vi "Draw Shapes.vi"(0 "Picture in":refnum<vi>, 1 "Commands":cluster{"Time (s)":dbl, T2, "Enabled":bool}[](array[cluster]), 3 "Sample Period (s)":dbl=0.02, 5 "Points":cluster{"x":dbl, "y":dbl, "th":dbl}[](array[cluster]), 6 "Path Points MEGA":cluster{"x":dbl, "y":dbl}[][](array[cluster]), 9 "new picture in":picture, 10 "Output Point MEGA":T1(array[cluster]), 11 "Results":T5, 12 "Output Point":T4, 14 "Path Points":cluster{"x":dbl, "y":dbl}[](array[cluster]), 15 "MEGA?":bool) -> (4 "new picture out":picture)   [LabVIEW 2023]
uses:
  Types/Single Cmd Info.ctl
  <vilib>/picture/picture.llb/imagedata.ctl
  Global Settings.vi
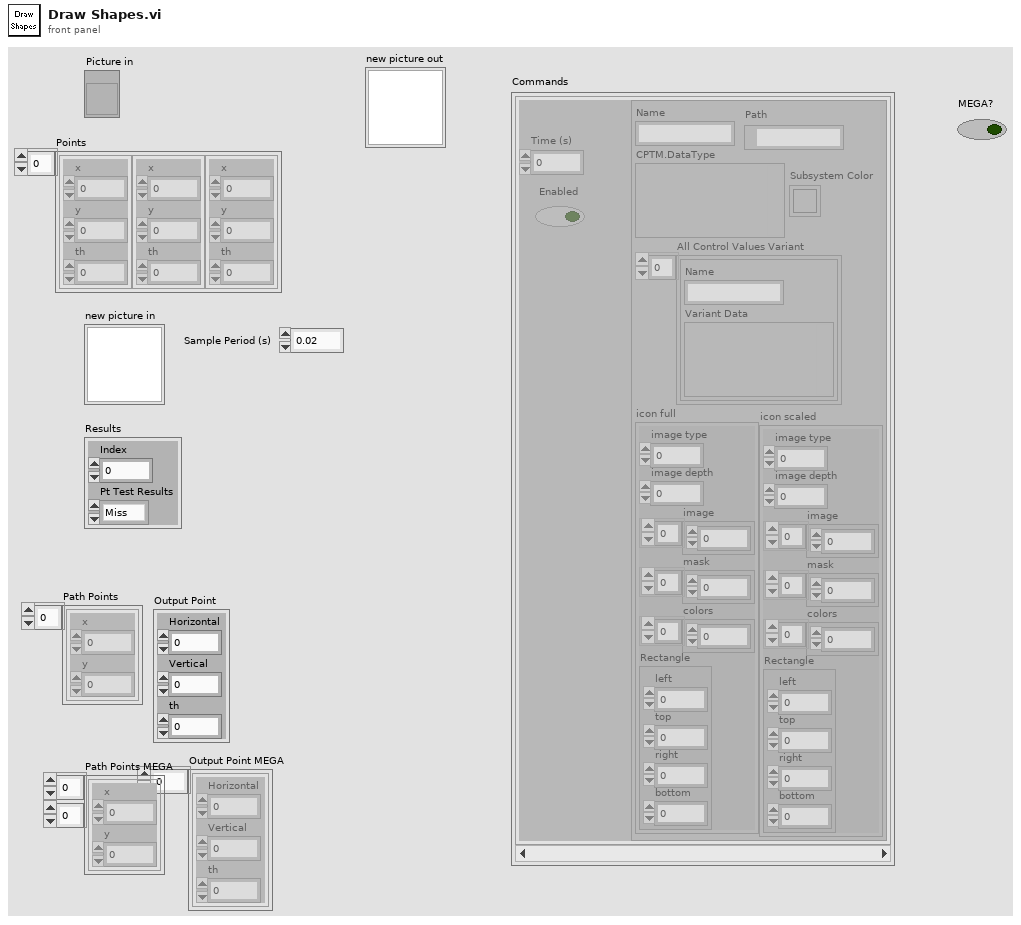
[diagram p1: front panel]
types:
  T1 = cluster{"Horizontal":dbl, "Vertical":dbl, "th":dbl}[]
  T2 = typedef "Single Cmd Info.ctl" = cluster{"Name":string, "CPTM.DataType":variant, "All Control Values Variant":cluster{"Name":string, "Variant Data":variant}[], "icon full":T3, "icon scaled":T3, "Path":path, "Subsystem Color":u32}
  T3 = typedef "imagedata.ctl" = cluster{"image type":i32, "image depth":i32, "image":u8[], "mask":u8[], "colors":u32[], "Rectangle":cluster{"left":i16, "top":i16, "right":i16, "bottom":i16}}
  T4 = cluster{"Horizontal":dbl, "Vertical":dbl, "th":dbl}
  T5 = cluster{"Index":i32, "Pt Test Results":enum16{"Miss", "Rect Hit", "Arrow Hit"}}
  T6 = typedef "LVPositionTypeDef.ctl" = cluster{"Left":i32, "Top":i32}
  T7 = typedef "LVBoundsTypeDef.ctl" = cluster{"Width":u32, "Height":u32}
  T8 = cluster{"left":i16, "top":i16, "right":i16, "bottom":i16}
  T9 = cluster{"Horizontal":dbl, "Vertical":dbl, "Horizontal":dbl, "Vertical":dbl}
  T10 = cluster{i32, "Pt Test Results":enum16{"Miss", "Rect Hit", "Arrow Hit"}}
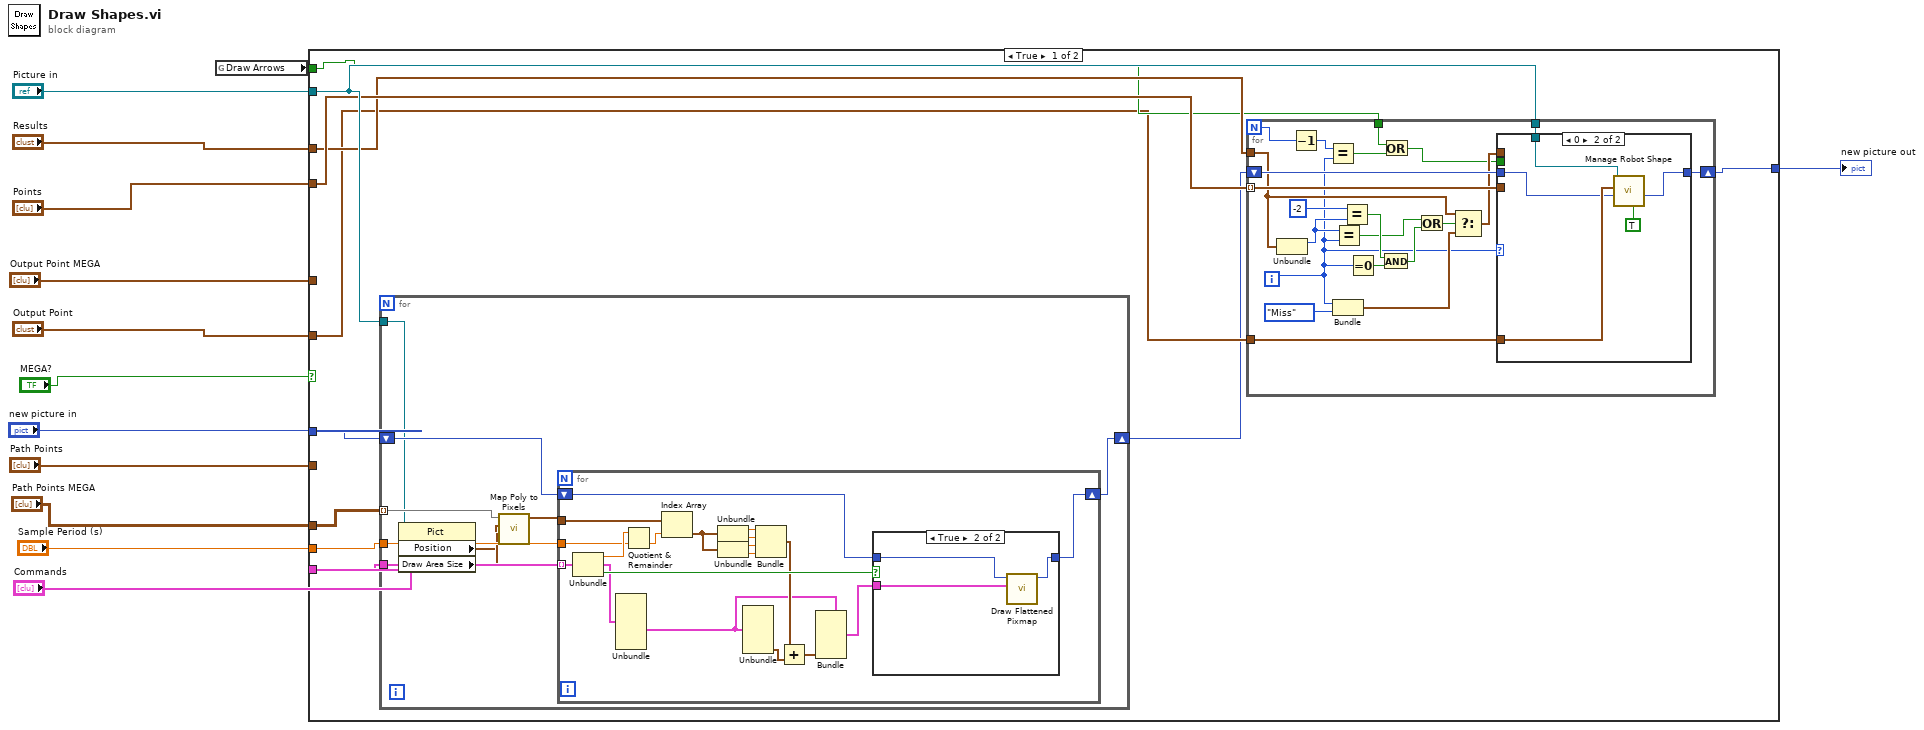
[diagram p0: block diagram]
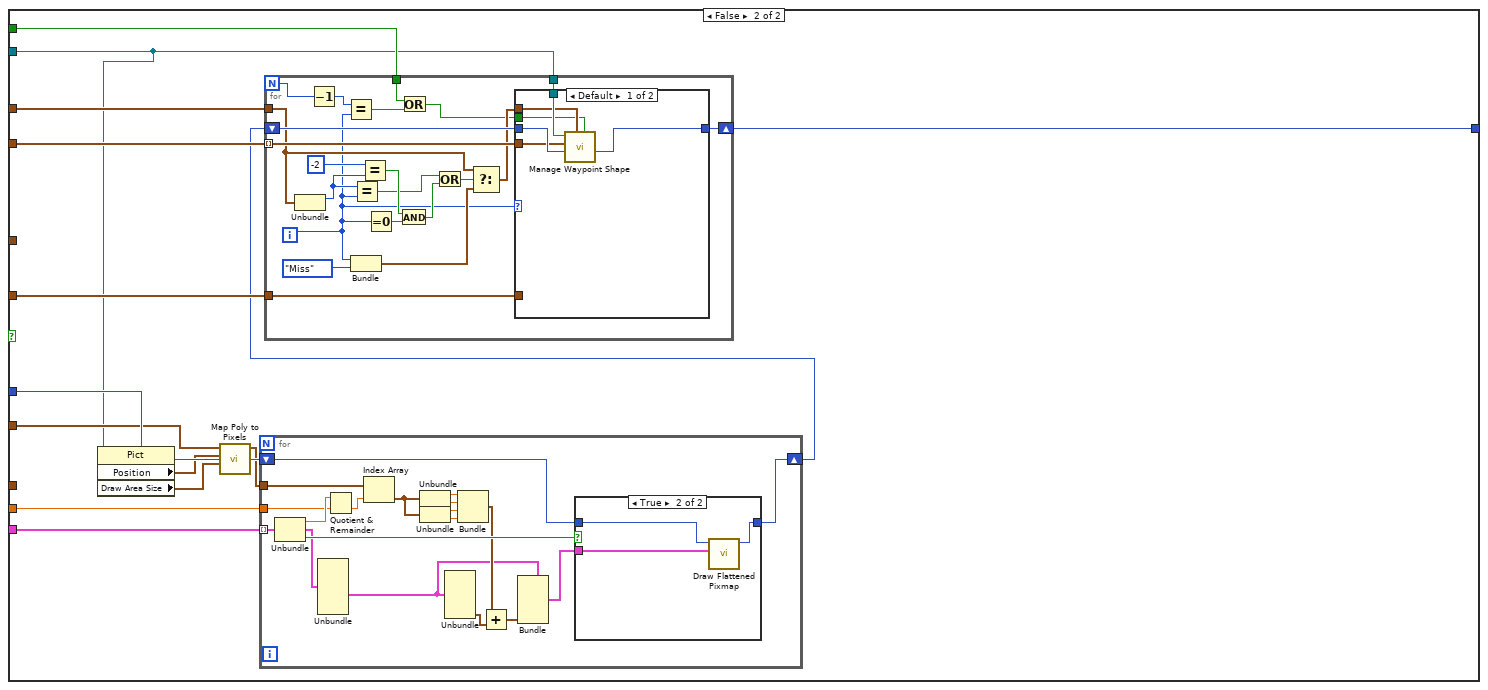
[diagram p4: hidden frame]
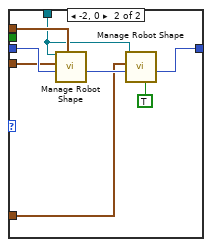
[diagram p6: hidden frame]
diagram:
  n1 = global read "Global Settings.vi" "Draw Arrows"() -> (w5:bool)
  n2 = case shown="True" "MEGA?" {
    tunnel: "Points" -> [w19 w98]
    tunnel: "Results" -> [w18 w97]
    tunnel: "Output Point" -> [w15 w96]
    tunnel: "Sample Period (s)" -> [w24 w95]
    tunnel: "Picture in" -> [w23 w86]
    tunnel: "Commands" -> [w22 w94]
    tunnel: "new picture in" -> [w21 w93]
    tunnel: [w16 w91] -> w6
    tunnel: w5 -> [w17 w90]
    tunnel: "Path Points" -> [_ w87]
    tunnel: "Path Points MEGA" -> [w20 _]
    tunnel: "Output Point MEGA" -> [_ _]
    frame True {
      n3 = for {
        tunnel: w24 -> [w61]
        tunnel: w23 -> [w54]
        tunnel: w20 -> [w55] mode=indexing
        tunnel: w22 -> [w60]
        shift-right: [w53] -> w14
        shift-left: w21 -> [w59]
        n4 = property on="Property Node" class="Pict"(reference=w54) -> ("Position"=w57:T6, "Draw Area Size"=w58:T7)  [unwired: 1 in, 2 out]
        n5 = call "Map Poly to Pixels.vi"("Draw Area Size"=w58, "Position"=w57, "Coords"=w55) -> ("Coords"=w56:cluster{"Horizontal":dbl, "Vertical":dbl}[])  [unwired: 8 in]
        n6 = for {
          shift-right: [w73] -> w53
          shift-left: w59 -> [w75]
          tunnel: w60 -> [w80] mode=indexing
          tunnel: w56 -> [w79]
          tunnel: w61 -> [w77]
          n7 = Unbundle(w80) -> ("Time (s)"=w78:dbl, w71:T2, "Enabled"=w74:bool)
          n8 = Unbundle(w71) -> ("icon scaled"=w63:T3)  [unwired: 6 out]
          n9 = Quotient & Remainder(x=w78, y=w77) -> (floor(x/y)=w76:dbl)  [unwired: 1 out]
          n10 = Index Array(array=w79, index=w76) -> (element=w62:cluster{"Horizontal":dbl, "Vertical":dbl})
          n11 = Unbundle(w62) -> ("Horizontal"=w70:dbl, "Vertical"=w69:dbl)
          n12 = Unbundle(w62) -> ("Horizontal"=w68:dbl, "Vertical"=w67:dbl)
          n13 = Unbundle(w63) -> ("Rectangle"=w65:T8)  [unwired: 5 out]
          n14 = Bundle("Horizontal"=w70, "Vertical"=w69, "Horizontal"=w68, "Vertical"=w67) -> (w64:T9)  [unwired: 1 in]
          n15 = Add(x=w64, y=w65) -> (x+y=w72:cluster{dbl, dbl, dbl, dbl})
          n16 = Bundle(cluster=w63, "Rectangle"=w72) -> (w66:T3)  [unwired: 5 in]
          n17 = case shown="True" w74 {
            tunnel: [w81 w82] -> w73
            tunnel: w75 -> [w81 w83]
            tunnel: w66 -> [_ w84]
            frame False {
            }
            frame True {
              n18 = call <vilib>:"Draw Flattened Pixmap.vi"("image data"=w84, "picture"=w83) -> ("new picture"=w82:picture)  [unwired: 7 in]
            }
          }
        }
      }
      n19 = for {
        N -> [w31]
        tunnel: w19 -> [w46] mode=indexing
        shift-right: [w45] -> w16
        shift-left: w14 -> [w44]
        tunnel: w23 -> [w43]
        tunnel: w18 -> [w40]
        tunnel: w15 -> [w28]
        tunnel: w17 -> [w25]
        i -> [w29]
        n20 = Unbundle(w40) -> ("Index"=w36:i32)  [unwired: 1 out]
        n21 = Decrement(x=w31) -> (x-1=w30:i32)
        n22 = Equal?(x=w30, y=w29) -> (x = y?=w27:bool)
        n23 = Bundle(w29, "Pt Test Results"=enum16{"Miss", "Rect Hit", "Arrow Hit"}."Miss") -> (w41:T10)  [unwired: 1 in]
        n24 = Equal?(x=w36, y=w29) -> (x = y?=w33:bool)
        n25 = Equal?(x=-2, y=w36) -> (x = y?=w35:bool)
        n26 = Equal To 0?(x=w29) -> (x = 0?=w38:bool)
        n27 = And(x=w35, y=w38) -> (x .and. y?=w34:bool)
        n28 = Or(x=w25, y=w27) -> (x .or. y?=w26:bool)
        n29 = Or(x=w33, y=w34) -> (x .or. y?=w32:bool)
        n30 = Select(t=w40, s=w32, f=w41) -> (s? t:f=w42:T5)
        n31 = case shown="0" w29 {
          tunnel: w46 -> [_ _]
          tunnel: [w47 w52] -> w45
          tunnel: w44 -> [w47 w48]
          tunnel: w43 -> [_ w50]
          tunnel: w42 -> [_ _]
          tunnel: w26 -> [_ _]
          tunnel: w28 -> [_ w51]
          frame Default {
          }
          frame 0 {
            n32 = call "Manage Robot Shape.vi"("Lighter"=TRUE ("Outline"), "new picture in"=w48, "Robot Position (ft)"=w51, "Pict Ref"=w50) -> ("new picture out"=w52:picture)  [unwired: 5 in, 2 out]
          }
        }
      }
    }
    frame False {
      n33 = property on="Property Node" class="Pict"(reference=w86) -> ("Position"=w89:T6, "Draw Area Size"=w88:T7)  [unwired: 1 in, 2 out]
      n34 = call "Map Poly to Pixels.vi"("Draw Area Size"=w88, "Position"=w89, "Coords"=w87) -> ("Coords"=w85:cluster{"Horizontal":dbl, "Vertical":dbl}[])  [unwired: 8 in]
      n35 = for {
        shift-right: [w110] -> w92
        shift-left: w93 -> [w112]
        tunnel: w94 -> [w117] mode=indexing
        tunnel: w85 -> [w116]
        tunnel: w95 -> [w114]
        n36 = Unbundle(w117) -> ("Time (s)"=w115:dbl, w108:T2, "Enabled"=w111:bool)
        n37 = Unbundle(w108) -> ("icon scaled"=w100:T3)  [unwired: 6 out]
        n38 = Quotient & Remainder(x=w115, y=w114) -> (floor(x/y)=w113:dbl)  [unwired: 1 out]
        n39 = Index Array(array=w116, index=w113) -> (element=w99:cluster{"Horizontal":dbl, "Vertical":dbl})
        n40 = Unbundle(w99) -> ("Horizontal"=w107:dbl, "Vertical"=w106:dbl)
        n41 = Unbundle(w99) -> ("Horizontal"=w105:dbl, "Vertical"=w104:dbl)
        n42 = Unbundle(w100) -> ("Rectangle"=w102:T8)  [unwired: 5 out]
        n43 = Bundle("Horizontal"=w107, "Vertical"=w106, "Horizontal"=w105, "Vertical"=w104) -> (w101:T9)  [unwired: 1 in]
        n44 = Add(x=w101, y=w102) -> (x+y=w109:cluster{dbl, dbl, dbl, dbl})
        n45 = Bundle(cluster=w100, "Rectangle"=w109) -> (w103:T3)  [unwired: 5 in]
        n46 = case shown="True" w111 {
          tunnel: [w118 w119] -> w110
          tunnel: w112 -> [w118 w120]
          tunnel: w103 -> [_ w121]
          frame False {
          }
          frame True {
            n47 = call <vilib>:"Draw Flattened Pixmap.vi"("image data"=w121, "picture"=w120) -> ("new picture"=w119:picture)  [unwired: 7 in]
          }
        }
      }
      n48 = for {
        N -> [w128]
        tunnel: w98 -> [w143] mode=indexing
        shift-right: [w142] -> w91
        shift-left: w92 -> [w141]
        tunnel: w86 -> [w140]
        tunnel: w97 -> [w137]
        tunnel: w96 -> [w125]
        tunnel: w90 -> [w122]
        i -> [w126]
        n49 = Unbundle(w137) -> ("Index"=w133:i32)  [unwired: 1 out]
        n50 = Decrement(x=w128) -> (x-1=w127:i32)
        n51 = Equal?(x=w127, y=w126) -> (x = y?=w124:bool)
        n52 = Bundle(w126, "Pt Test Results"=enum16{"Miss", "Rect Hit", "Arrow Hit"}."Miss") -> (w138:T10)  [unwired: 1 in]
        n53 = Equal?(x=w133, y=w126) -> (x = y?=w130:bool)
        n54 = Equal?(x=-2, y=w133) -> (x = y?=w132:bool)
        n55 = Equal To 0?(x=w126) -> (x = 0?=w135:bool)
        n56 = And(x=w132, y=w135) -> (x .and. y?=w131:bool)
        n57 = Or(x=w122, y=w124) -> (x .or. y?=w123:bool)
        n58 = Or(x=w130, y=w131) -> (x .or. y?=w129:bool)
        n59 = Select(t=w137, s=w129, f=w138) -> (s? t:f=w139:T5)
        n60 = case shown="Default" w126 {
          tunnel: w143 -> [w145 w156]
          tunnel: [w148 w153] -> w142
          tunnel: w141 -> [w149 w157]
          tunnel: w140 -> [w147 w151]
          tunnel: w139 -> [w146 w155]
          tunnel: w123 -> [w144 _]
          tunnel: w125 -> [_ w152]
          frame Default {
            n61 = call "Manage Waypoint Shape.vi"("Draw Arrow"=w144, "Drawing Options"=w146, "new picture in"=w149, "Waypoint Position (ft)"=w145, "Pict Ref"=w147) -> ("new picture out"=w148:picture)  [unwired: 5 in, 1 out]
          }
          frame -2, 0 {
            n62 = call "Manage Robot Shape.vi"("Drawing Options"=w155, "new picture in"=w157, "Robot Position (ft)"=w156, "Pict Ref"=w151) -> ("new picture out"=w154:picture)  [unwired: 5 in, 2 out]
            n63 = call "Manage Robot Shape.vi"("Lighter"=TRUE ("Outline"), "new picture in"=w154, "Robot Position (ft)"=w152, "Pict Ref"=w151) -> ("new picture out"=w153:picture)  [unwired: 5 in, 2 out]
          }
        }
      }
    }
  }
  "new picture out" <- w6
